vi "Start Inline Receive.vi"(8 "error in (no error)":errorcluster, 11 "Framework in":refnum<class "Framework.lvclass">) -> (0 "error out":errorcluster, 3 "Framework out":refnum<class "Framework.lvclass">)   [LabVIEW 2017, in "Data Sharing Framework Core.lvlib" / "Data Sharing Framework Engine.lvlib" / "Framework.lvclass"]
uses:
  Framework.lvclass
  Framework.lvclass/Framework.ctl
  Plugin/Plugin.lvclass/Plugin.ctl
  Internal/Timing/Engine Timing.lvclass/Engine Timing.ctl
  Transfer Group/Transfer Group.lvclass/Transfer Group.ctl
  Transfer Group/Increment Iteration.vi
  Plugin/Get Timing.vi
  Internal/Timing/Is Active Cycle.vi
  Internal/Timing/Increment Iteration Count.vi
  Internal/Timing/Get Decimation.vi
  Internal/Timing/Get Offset.vi
  Internal/Interfaces/Transceiver Interface/Write Command to Transfer Group.vi
  Plugin/Obtain Transceiver Thread.vi
  Plugin/Plugin.lvclass
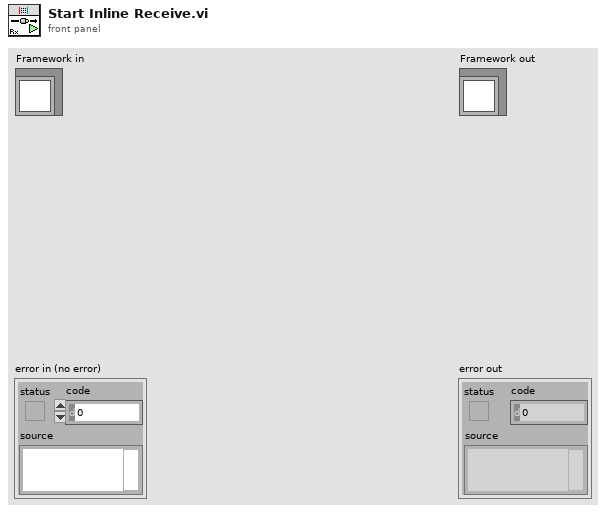
[diagram p1: front panel]
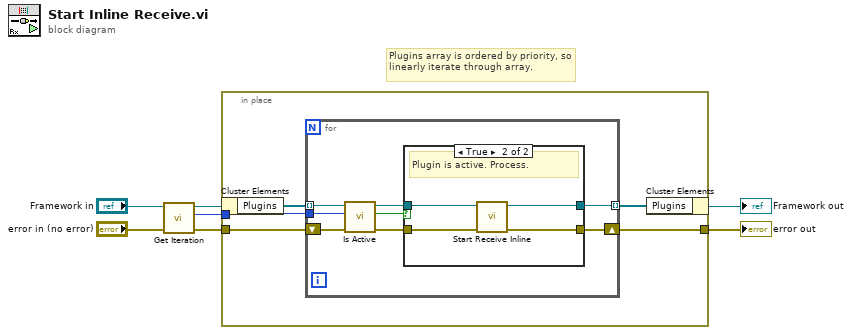
[diagram p0: block diagram]
diagram:
  # "Plugins array is ordered by priority, so linearly iterate through array."
  n1 = call "Get Iteration.vi"("Framework in"="Framework in") -> ("iteration"=w4:u64, "Framework out"=w1:refnum<class "Framework.lvclass">)  [unwired: 9 in]
  n2 = in-place {
    in-place-border: "error in (no error)" -> [w11]
    in-place-border: [w10] -> w5
    in-place-border: w4 -> [w9]
    n3 = in-place-cluster #1(w1) -> ("Plugins"=w8:refnum<class "Plugin.lvclass">[])
    n4 = for {
      tunnel: w8 -> [w12] mode=indexing
      tunnel: [w18] -> w7 mode=indexing
      shift-right: [w17] -> w10
      shift-left: w11 -> [w16]
      tunnel: w9 -> [w14]
      n5 = call "Is Active.vi"("cycle count"=w14, "Plugin in"=w12) -> ("active this cycle?"=w13:bool, "Plugin out"=w15:refnum<class "Plugin.lvclass">)  [unwired: 8 in]
      n6 = case shown="True" w13 {
        tunnel: w15 -> [w20 w24]
        tunnel: [w20 w23] -> w18
        tunnel: [w19 w21] -> w17
        tunnel: w16 -> [w19 w22]
        frame False {
          # "Plugin is not active. Skip."
        }
        frame True {
          # "Plugin is active. Process."
          n7 = call "Start Receive Inline.vi"("error in (no error)"=w22, "Plugin in"=w24) -> ("error out"=w21:errorcluster, "Plugin out"=w23:refnum<class "Plugin.lvclass">)  [unwired: 8 in]
        }
      }
    }
    n8 = in-place-cluster #1("Plugins"=w7) -> (→"Framework out":refnum<class "Framework.lvclass">)
  }
  "error out" <- w5
